vi "Set (U32).vi"(9 "Value":u32, 10 "Key":string, 11 "Dictionary in":variant) -> (2 "replaced":bool, 3 "Dictionary out":variant)   [LabVIEW 2011, in "Dictionary.lvlib"]
doc: "Sets (Add or Replace) a value in the dictionary with passed in key and value."
uses:
  Dictionary.lvlib
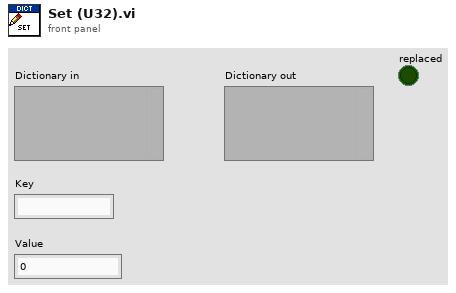
[diagram p1: front panel]
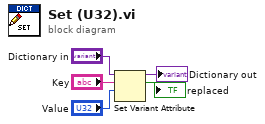
[diagram p0: block diagram]
diagram:
  n1 = Set Variant Attribute(Variant="Dictionary in", name="Key", value="Value") -> (Variant out=→"Dictionary out":variant, replaced=→"replaced":bool)  [unwired: 1 in, 1 out]
